vi "Init Communication.vi"(8 "error in (no error)":errorcluster, 10 "Async Data in":T1, 11 "Async Input in":T4={"Device Ref"=18446744073709551615, "Waveforms"=[], "Channels"={"Command Chan Refs"=[], "Command Data Refs"=[], "Command Values"=[], "Status Chan Refs"=[], "Status Data Refs"=[], "Status Values"=[], "System Time"={"System Time"=timestamp(0 s since 1904-01-01), "Data Reference"=0, "Absolute Time Channel Data Ref"=0, "Get Date-Time Channel Data Ref"=0}, "Trigger Chan Refs"=[], "Trigger Data Refs"=[], "Trigger Values"=[]}, "Waveform Logs"=[], "Communication"={"Async Status"=refnum, "Wfm Comm Properties"={"WPL"={"Custom Queue Size"=1, "Use Custom Queue Size?"=FALSE}}, "Shutdown Event"=refnum, "Trigger Event"=refnum, "New File Event"=refnum, "Log Queues"=[], "Async VI Ref"=refnum}, "error"={"status"=FALSE, "code"=0, "source"=""}} {"Device Ref" format="%.0x"; "Channels"."Trigger Data Refs"."Data Reference" format="%.0x"; "Channels"."Trigger Chan Refs" format="%.0x"; "Channels"."System Time"."Get Date-Time Channel Data Ref" format="%.0x"; "Channels"."System Time"."Absolute Time Channel Data Ref" format="%.0x"; "Channels"."System Time"."Channel Data Reference" format="%.0x"; "Channels"."Status Data Refs"."Data Reference" format="%.0x"; "Channels"."Command Data Refs"."Data Reference" format="%.0x"; "Channels"."Status Chan Refs" format="%.0x"; "Channels"."Command Chan Refs" format="%.0x"; "Waveforms"."Waveform Ref in" format="%.0x"; "Waveform Logs"."Node ID" format="%.0x"; "Waveform Logs"."TDMS Error Code"."Data Ref" format="%.0x"; "Waveform Logs"."Missed Samples"."Data Ref" format="%.0x"; "Waveform Logs"."File Status"."Data Ref" format="%.0x"; "Waveform Logs"."Start New File"."Data Ref" format="%.0x"; "Waveform Logs"."Logging Enabled"."Data Ref" format="%.0x"; "Waveform Logs"."Stop Trigger"."Node Data Ref" format="%.0x"; "Waveform Logs"."Stop Trigger"."Node ID" format="%.0x"; "Waveform Logs"."Start Trigger"."Node Data Ref" format="%.0x"; "Waveform Logs"."Start Trigger"."Node ID" format="%.0x"}) -> (0 "error out":errorcluster, 1 "Event Registration":refnum<event-registration>, 2 "Async Data out":T1, 3 "Async Input out":T4={"Device Ref"=18446744073709551615, "Waveforms"=[], "Channels"={"Command Chan Refs"=[], "Command Data Refs"=[], "Command Values"=[], "Status Chan Refs"=[], "Status Data Refs"=[], "Status Values"=[], "System Time"={"System Time"=timestamp(0 s since 1904-01-01), "Data Reference"=0, "Absolute Time Channel Data Ref"=0, "Get Date-Time Channel Data Ref"=0}, "Trigger Chan Refs"=[], "Trigger Data Refs"=[], "Trigger Values"=[]}, "Waveform Logs"=[], "Communication"={"Async Status"=refnum, "Wfm Comm Properties"={"WPL"={"Custom Queue Size"=1, "Use Custom Queue Size?"=FALSE}}, "Shutdown Event"=refnum, "Trigger Event"=refnum, "New File Event"=refnum, "Log Queues"=[], "Async VI Ref"=refnum}, "error"={"status"=FALSE, "code"=0, "source"=""}} {"Device Ref" format="%.0x"; "Channels"."Trigger Data Refs"."Data Reference" format="%.0x"; "Channels"."Trigger Chan Refs" format="%.0x"; "Channels"."System Time"."Get Date-Time Channel Data Ref" format="%.0x"; "Channels"."System Time"."Absolute Time Channel Data Ref" format="%.0x"; "Channels"."System Time"."Channel Data Reference" format="%.0x"; "Channels"."Status Data Refs"."Data Reference" format="%.0x"; "Channels"."Command Data Refs"."Data Reference" format="%.0x"; "Channels"."Status Chan Refs" format="%.0x"; "Channels"."Command Chan Refs" format="%.0x"; "Waveforms"."Waveform Ref in" format="%.0x"; "Waveform Logs"."Node ID" format="%.0x"; "Waveform Logs"."TDMS Error Code"."Data Ref" format="%.0x"; "Waveform Logs"."Missed Samples"."Data Ref" format="%.0x"; "Waveform Logs"."File Status"."Data Ref" format="%.0x"; "Waveform Logs"."Start New File"."Data Ref" format="%.0x"; "Waveform Logs"."Logging Enabled"."Data Ref" format="%.0x"; "Waveform Logs"."Stop Trigger"."Node Data Ref" format="%.0x"; "Waveform Logs"."Stop Trigger"."Node ID" format="%.0x"; "Waveform Logs"."Start Trigger"."Node Data Ref" format="%.0x"; "Waveform Logs"."Start Trigger"."Node ID" format="%.0x"})   [LabVIEW 2015, in "Waveform Data Logger Engine.lvlib"]
uses:
  Waveform Data Logger Engine.lvlib
  Types/RT Data.ctl
  <vilib>/NI Veristand/Custom Device API/Custom Device Item Ref.ctl
  Types/Inline Waveform Info.ctl
  <vilib>/NI Veristand/Custom Device API/Waveform Data Reference.ctl
  Classes/Waveforms/Waveform Receive/Associated Log.ctl
  <vilib>/NI Veristand/Custom Device API/Custom Device Waveform DataType.ctl
  Types/Channels.ctl
  <vilib>/NI Veristand/Custom Device API/Block Data Reference.ctl
  <vilib>/NI Veristand/Custom Device API/Data Reference.ctl
  Types/System Time.ctl
  Types/Inline Waveform Log Info.ctl
  Classes/Log File Specifications/Waveform TDMS Log File Specification/Waveform TDMS Log File Specification.lvclass
  Classes/Triggers/Trigger/Trigger.lvclass
  Types/Inline Log Waveform.ctl
  Types/Trigger Settings.ctl
  Types/Log Status.ctl
  Types/Channel.ctl
  Types/Communication.ctl
  Types/Async Status.ctl
  Types/Async State.ctl
  <vilib>/NI Veristand/Custom Device Waveform API/Communication Properties.ctl
  Types/Trigger Event Data.ctl
  Types/Trigger Received.ctl
  Types/New File Event Data.ctl
  Types/Log Queues.ctl
  Types/Async Data.ctl
  <vilib>/NI VeriStand/Custom Device Waveform API/Multiple Waveforms Read (DBL)/Multiple Waveforms Read (DBL).lvclass
  Classes/Waveforms/Utilities/Reference Dictionary/Reference Dictionary.lvclass
  Types/Wfm Acq Data.ctl
  Classes/Waveforms/Waveform Receive/Waveform Receive.lvclass
  Classes/Waveforms/Waveform Log/Waveform Log.lvclass
  Types/Async Communication.ctl
  Types/Check File Loop Cmd.ctl
  <vilib>/NI Veristand/Custom Device API/Custom Device API.lvlib
  <vilib>/NI Veristand/Custom Device Waveform API/NI_VS Custom Device Waveform API.lvlib
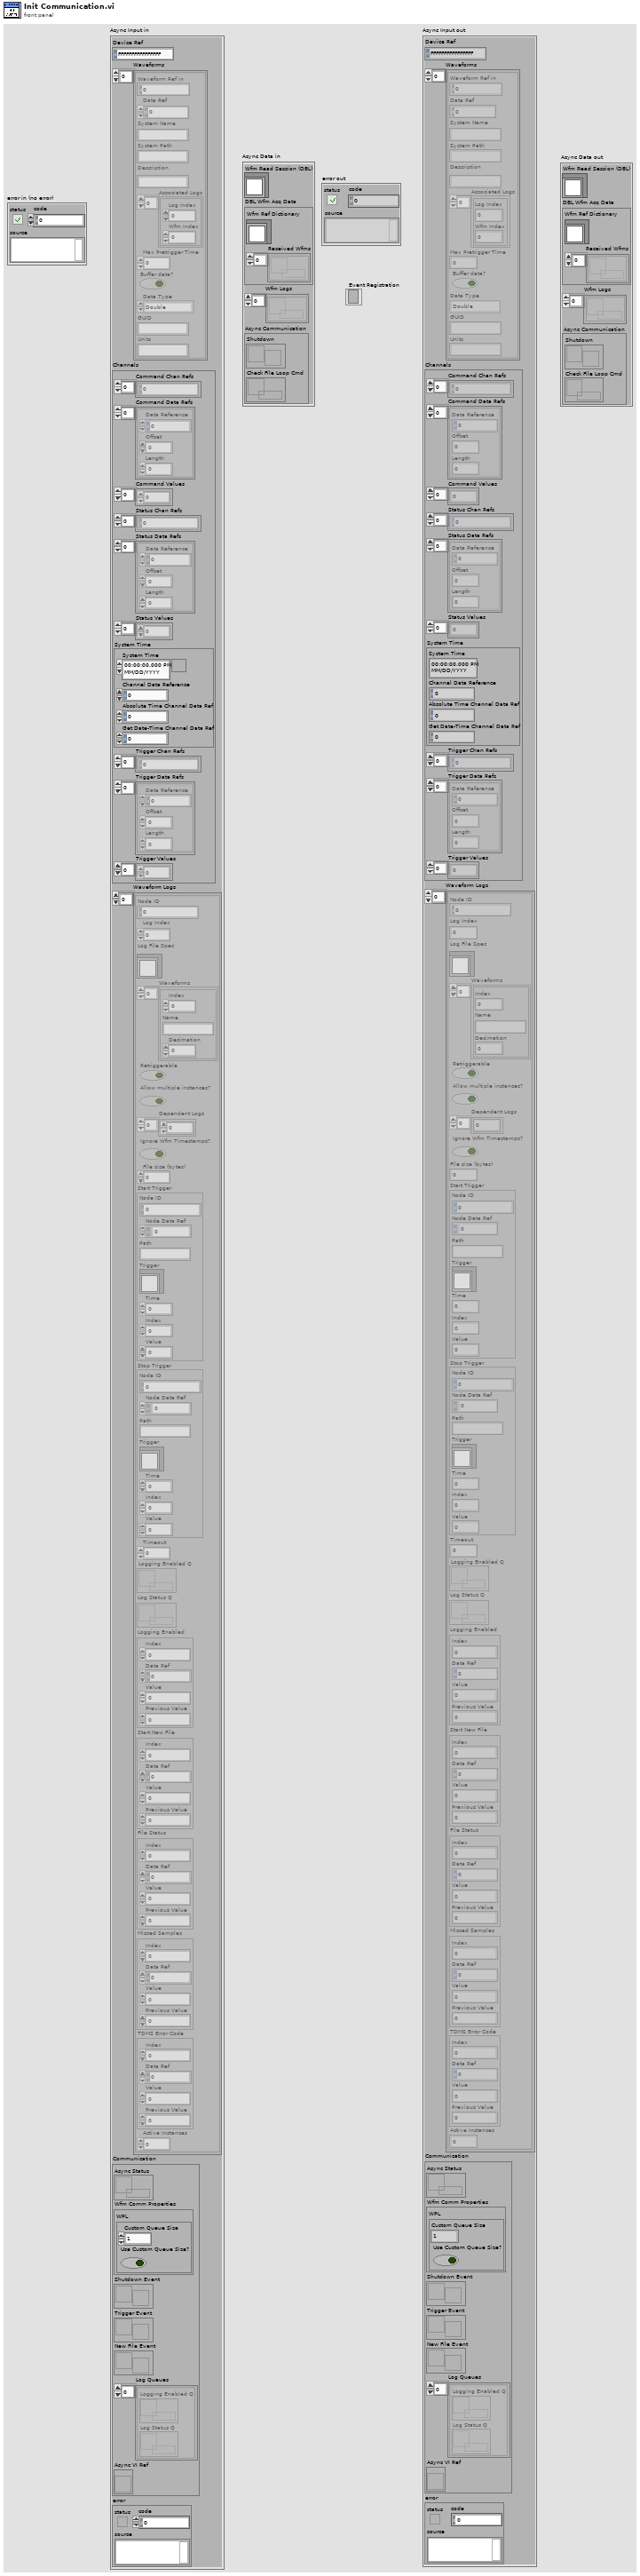
[diagram p1: front panel]
types:
  T1 = typedef "Waveform Data Logger Engine.lvlib/Async Data.ctl" = cluster{"Wfm Read Session (DBL)":refnum<class "Multiple Waveforms Read (DBL).lvclass">, "DBL Wfm Acq Data":T2, "Wfm Logs":refnum<data-value>[], "Async Communication":T3}
  T2 = typedef "Waveform Data Logger Engine.lvlib/Wfm Acq Data.ctl" = cluster{"Wfm Ref Dictionary":refnum<class "Reference Dictionary.lvclass">, "Received Wfms":refnum<data-value>[]}
  T3 = typedef "Waveform Data Logger Engine.lvlib/Async Communication.ctl" = cluster{"Shutdown":refnum<user-event>, "Check File Loop Cmd":refnum<queue>}
  T4 = typedef "Waveform Data Logger Engine.lvlib/RT Data.ctl" = cluster{"Device Ref":T5, "Waveforms":T6[], "Channels":T10, "Waveform Logs":T14[], "Communication":T18, "error":errorcluster}
  T5 = typedef "Custom Device API.lvlib/Custom Device Item Ref.ctl" = u64
  T6 = typedef "Waveform Data Logger Engine.lvlib/Inline Waveform Info.ctl" = cluster{"Waveform Ref in":T5, "Data Ref":T7, "System Name":string, "System Path":string, "Description":string, "Associated Logs":T8[], "Max Pretrigger Time":dbl, "Buffer data?":bool, "Data Type":T9, "GUID":string, "Units":string}
  T7 = typedef "Custom Device API.lvlib/Waveform Data Reference.ctl" = i32
  T8 = typedef "Waveform Receive.lvclass/Associated Log.ctl" = cluster{"Log Index":i32, "Wfm Index":i32}
  T9 = typedef "Custom Device API.lvlib/Custom Device Waveform DataType.ctl" = enum16{"Double", "Complex Double"}
  T10 = typedef "Waveform Data Logger Engine.lvlib/Channels.ctl" = cluster{"Command Chan Refs":T5[], "Command Data Refs":T11[], "Command Values":dbl[], "Status Chan Refs":T5[], "Status Data Refs":T11[], "Status Values":dbl[], "System Time":T13, "Trigger Chan Refs":T5[], "Trigger Data Refs":T11[], "Trigger Values":dbl[]}
  T11 = typedef "Custom Device API.lvlib/Block Data Reference.ctl" = cluster{"Data Reference":T12, "Offset":u64, "Length":u64}
  T12 = typedef "Custom Device API.lvlib/Data Reference.ctl" = i32
  T13 = typedef "Waveform Data Logger Engine.lvlib/System Time.ctl" = cluster{"System Time":timestamp, "Data Reference":T12, "Absolute Time Channel Data Ref":T12, "Get Date-Time Channel Data Ref":T12}
  T14 = typedef "Waveform Data Logger Engine.lvlib/Inline Waveform Log Info.ctl" = cluster{"Node ID":T5, "Log Index":i32, "Log File Spec":refnum<class "Waveform TDMS Log File Specification.lvclass">, "Waveforms":T15[], "Retriggerable":bool, "Allow multiple instances?":bool, "Dependent Logs":i32[], "Ignore Wfm Timestamps?":bool, "File size (bytes)":i64, "Start Trigger":T16, "Stop Trigger":T16, "Timeout":dbl, "Logging Enabled Q":refnum<queue>, "Log Status Q":refnum<queue>, "Logging Enabled":T17, "Start New File":T17, "File Status":T17, "Missed Samples":T17, "TDMS Error Code":T17, "Active Instances":i32}
  T15 = typedef "Waveform Data Logger Engine.lvlib/Inline Log Waveform.ctl" = cluster{"Index":i32, "Name":string, "Decimation":u32}
  T16 = typedef "Waveform Data Logger Engine.lvlib/Trigger Settings.ctl" = cluster{"Node ID":T5, "Node Data Ref":i32, "Path":string, "Trigger":refnum<class "Trigger.lvclass">, "Time":dbl, "Index":i32, "Value":dbl}
  T17 = typedef "Waveform Data Logger Engine.lvlib/Channel.ctl" = cluster{"Index":i32, "Data Ref":T12, "Value":dbl, "Previous Value":dbl}
  T18 = typedef "Waveform Data Logger Engine.lvlib/Communication.ctl" = cluster{"Async Status":refnum<queue>, "Wfm Comm Properties":T19, "Shutdown Event":refnum<user-event>, "Trigger Event":refnum<user-event>, "New File Event":refnum<user-event>, "Log Queues":T20[], "Async VI Ref":refnum<vi>}
  T19 = typedef "NI_VS Custom Device Waveform API.lvlib/Communication Properties.ctl" = cluster{"WPL":cluster{"Custom Queue Size":i32, "Use Custom Queue Size?":bool}}
  T20 = typedef "Waveform Data Logger Engine.lvlib/Log Queues.ctl" = cluster{"Logging Enabled Q":refnum<queue>, "Log Status Q":refnum<queue>}
  T21 = typedef "Waveform Data Logger Engine.lvlib/Check File Loop Cmd.ctl" = enum16{"None", "Stop"}
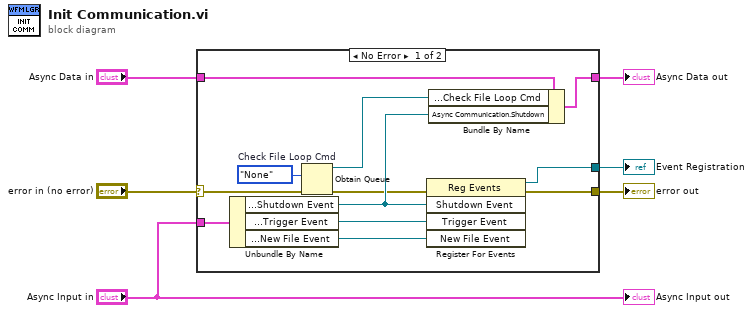
[diagram p0: block diagram]
diagram:
  n1 = case shown="No Error" "error in (no error)" {
    selector: "error in (no error)" -> [w9 w20]
    tunnel: [w11 w20] -> w5
    tunnel: "Async Data in" -> [w14 w19]
    tunnel: [w13 w19] -> w4
    tunnel: "Async Input in" -> [w15 _]
    tunnel: [w12 _] -> w1
    frame No Error {
      w10 = Check_File_Loop_Cmd."None"  # Check File Loop Cmd
      n2 = Unbundle By Name(w15) -> ("Communication.Shutdown Event"=w16:refnum<user-event>, "Communication.Trigger Event"=w17:refnum<user-event>, "Communication.New File Event"=w18:refnum<user-event>)
      n3 = Obtain Queue(element data type=w10, error in (no error)=w9) -> (queue out=w7:refnum<queue>, error out=w8:errorcluster)  [unwired: 3 in, 1 out]
      n4 = register-events(error in=w8, w16, w17, w18) -> (reference out=w12:refnum<event-registration>, error out=w11:errorcluster)  [unwired: 1 in]
      n5 = Bundle By Name(cluster=w14, "Async Communication.Check File Loop Cmd"=w7, "Async Communication.Shutdown"=w16) -> (w13:T1)
    }
    frame Error {
    }
  }
  "Async Data out" <- w4
  "error out" <- w5
  "Event Registration" <- w1
  "Async Input out" <- "Async Input in"
